vi "FipsAdjacent.vi"() -> (11 "Fips":i32[](array[numeric]))   [LabVIEW 2017] (continued)
\"\t36077\t\"Madison County, NY\"\t36053\n\"Otsego County, NY\"\t36077\t\"Montgomery County, NY\"\t36057\n\"Otsego County, NY\"\t36077\t\"Oneida County, NY\"\t36065\n\"Otsego County, NY\"\t36077\t\"Otsego County, NY\"\t36077\n\"Otsego County, NY\"\t36077\t\"Schoharie County, NY\"\t36095\n\"Putnam County, NY\"\t36079\t\"Fairfield County, CT\"\t09001\n\"Putnam County, NY\"\t36079\t\"Dutchess County, NY\"\t36027\n\"Putnam County, NY\"\t36079\t\"Orange County, NY\"\t36071\n\"Putnam County, NY\"\t36079\t\"Putnam County, NY\"\t36079\n\"Putnam County, NY\"\t36079\t\"Rockland County, NY\"\t36087\n\"Putnam County, NY\"\t36079\t\"Westchester County, NY\"\t36119\n\"Queens County, NY\"\t36081\t\"Monmouth County, NJ\"\t34025\n\"Queens County, NY\"\t36081\t\"Bronx County, NY\"\t36005\n\"Queens County, NY\"\t36081\t\"Kings County, NY\"\t36047\n\"Queens County, NY\"\t36081\t\"Nassau County, NY\"\t36059\n\"Queens County, NY\"\t36081\t\"New York County, NY\"\t36061\n\"Queens County, NY\"\t36081\t\"Queens County, NY\"\t36081\n\"Queens County, NY\"\t36081\t\"Richmond County, NY\"\t36085\n\"Rensselaer County, NY\"\t36083\t\"Berkshire County, MA\"\t25003\n\"Rensselaer County, NY\"\t36083\t\"Albany County, NY\"\t36001\n\"Rensselaer County, NY\"\t36083\t\"Columbia County, NY\"\t36021\n\"Rensselaer County, NY\"\t36083\t\"Greene County, NY\"\t36039\n\"Rensselaer County, NY\"\t36083\t\"Rensselaer County, NY\"\t36083\n\"Rensselaer County, NY\"\t36083\t\"Saratoga County, NY\"\t36091\n\"Rensselaer County, NY\"\t36083\t\"Washington County, NY\"\t36115\n\"Rensselaer County, NY\"\t36083\t\"Bennington County, VT\"\t50003\n\"Richmond County, NY\"\t36085\t\"Hudson County, NJ\"\t34017\n\"Richmond County, NY\"\t36085\t\"Middlesex County, NJ\"\t34023\n\"Richmond County, NY\"\t36085\t\"Monmouth County, NJ\"\t34025\n\"Richmond County, NY\"\t36085\t\"Union County, NJ\"\t34039\n\"Richmond County, NY\"\t36085\t\"Kings County, NY\"\t36047\n\"Richmond County, NY\"\t36085\t\"Queens County, NY\"\t36081\n\"Richmond County, NY\"\t36085\t\"Richmond County, NY\"\t36085\n\"Rockland County, NY\"\t36087\t\"Bergen County, NJ\"\t34003\n\"Rockland County, NY\"\t36087\t\"Passaic County, NJ\"\t34031\n\"Rockland County, NY\"\t36087\t\"Orange County, NY\"\t36071\n\"Rockland County, NY\"\t36087\t\"Putnam County, NY\"\t36079\n\"Rockland County, NY\"\t36087\t\"Rockland County, NY\"\t36087\n\"Rockland County, NY\"\t36087\t\"Westchester County, NY\"\t36119\n\"St. Lawrence County, NY\"\t36089\t\"Franklin County, NY\"\t36033\n\"St. Lawrence County, NY\"\t36089\t\"Hamilton County, NY\"\t36041\n\"St. Lawrence County, NY\"\t36089\t\"Herkimer County, NY\"\t36043\n\"St. Lawrence County, NY\"\t36089\t\"Jefferson County, NY\"\t36045\n\"St. Lawrence County, NY\"\t36089\t\"Lewis County, NY\"\t36049\n\"St. Lawrence County, NY\"\t36089\t\"St. Lawrence County, NY\"\t36089\n\"Saratoga County, NY\"\t36091\t\"Albany County, NY\"\t36001\n\"Saratoga County, NY\"\t36091\t\"Fulton County, NY\"\t36035\n\"Saratoga County, NY\"\t36091\t\"Hamilton County, NY\"\t36041\n\"Saratoga County, NY\"\t36091\t\"Montgomery County, NY\"\t36057\n\"Saratoga County, NY\"\t36091\t\"Rensselaer County, NY\"\t36083\n\"Saratoga County, NY\"\t36091\t\"Saratoga County, NY\"\t36091\n\"Saratoga County, NY\"\t36091\t\"Schenectady County, NY\"\t36093\n\"Saratoga County, NY\"\t36091\t\"Warren County, NY\"\t36113\n\"Saratoga County, NY\"\t36091\t\"Washington County, NY\"\t36115\n\"Schenectady County, NY\"\t36093\t\"Albany County, NY\"\t36001\n\"Schenectady County, NY\"\t36093\t\"Montgomery County, NY\"\t36057\n\"Schenectady County, NY\"\t36093\t\"Saratoga County, NY\"\t36091\n\"Schenectady County, NY\"\t36093\t\"Schenectady County, NY\"\t36093\n\"Schenectady County, NY\"\t36093\t\"Schoharie County, NY\"\t36095\n\"Schoharie County, NY\"\t36095\t\"Albany County, NY\"\t36001\n\"Schoharie County, NY\"\t36095\t\"Delaware County, NY\"\t36025\n\"Schoharie County, NY\"\t36095\t\"Greene County, NY\"\t36039\n\"Schoharie County, NY\"\t36095\t\"Montgomery County, NY\"\t36057\n\"Schoharie County, NY\"\t36095\t\"Otsego County, NY\"\t36077\n\"Schoharie County, NY\"\t36095\t\"Schenectady County, NY\"\t36093\n\"Schoharie County, NY\"\t36095\t\"Schoharie County, NY\"\t36095\n\"Schuyler County, NY\"\t36097\t\"Chemung County, NY\"\t36015\n\"Schuyler County, NY\"\t36097\t\"Schuyler County, NY\"\t36097\n\"Schuyler County, NY\"\t36097\t\"Seneca County, NY\"\t36099\n\"Schuyler County, NY\"\t36097\t\"Steuben County, NY\"\t36101\n\"Schuyler County, NY\"\t36097\t\"Tompkins County, NY\"\t36109\n\"Schuyler County, NY\"\t36097\t\"Yates County, NY\"\t36123\n\"Seneca County, NY\"\t36099\t\"Cayuga County, NY\"\t36011\n\"Seneca County, NY\"\t36099\t\"Ontario County, NY\"\t36069\n\"Seneca County, NY\"\t36099\t\"Schuyler County, NY\"\t36097\n\"Seneca County, NY\"\t36099\t\"Seneca County, NY\"\t36099\n\"Seneca County, NY\"\t36099\t\"Tompkins County, NY\"\t36109\n\"Seneca County, NY\"\t36099\t\"Wayne County, NY\"\t36117\n\"Seneca County, NY\"\t36099\t\"Yates County, NY\"\t36123\n\"Steuben County, NY\"\t36101\t\"Allegany County, NY\"\t36003\n\"Steuben County, NY\"\t36101\t\"Chemung County, NY\"\t36015\n\"Steuben County, NY\"\t36101\t\"Livingston County, NY\"\t36051\n\"Steuben County, NY\"\t36101\t\"Ontario County, NY\"\t36069\n\"Steuben County, NY\"\t36101\t\"Schuyler County, NY\"\t36097\n\"Steuben County, NY\"\t36101\t\"Steuben County, NY\"\t36101\n\"Steuben County, NY\"\t36101\t\"Yates County, NY\"\t36123\n\"Steuben County, NY\"\t36101\t\"Potter County, PA\"\t42105\n\"Steuben County, NY\"\t36101\t\"Tioga County, PA\"\t42117\n\"Suffolk County, NY\"\t36103\t\"Fairfield County, CT\"\t09001\n\"Suffolk County, NY\"\t36103\t\"Middlesex County, CT\"\t09007\n\"Suffolk County, NY\"\t36103\t\"New Haven County, CT\"\t09009\n\"Suffolk County, NY\"\t36103\t\"New London County, CT\"\t09011\n\"Suffolk County, NY\"\t36103\t\"Nassau County, NY\"\t36059\n\"Suffolk County, NY\"\t36103\t\"Suffolk County, NY\"\t36103\n\"Suffolk County, NY\"\t36103\t\"Washington County, RI\"\t44009\n\"Sullivan County, NY\"\t36105\t\"Delaware County, NY\"\t36025\n\"Sullivan County, NY\"\t36105\t\"Orange County, NY\"\t36071\n\"Sullivan County, NY\"\t36105\t\"Sullivan County, NY\"\t36105\n\"Sullivan County, NY\"\t36105\t\"Ulster County, NY\"\t36111\n\"Sullivan County, NY\"\t36105\t\"Pike County, PA\"\t42103\n\"Sullivan County, NY\"\t36105\t\"Wayne County, PA\"\t42127\n\"Tioga County, NY\"\t36107\t\"Broome County, NY\"\t36007\n\"Tioga County, NY\"\t36107\t\"Chemung County, NY\"\t36015\n\"Tioga County, NY\"\t36107\t\"Cortland County, NY\"\t36023\n\"Tioga County, NY\"\t36107\t\"Tioga County, NY\"\t36107\n\"Tioga County, NY\"\t36107\t\"Tompkins County, NY\"\t36109\n\"Tioga County, NY\"\t36107\t\"Bradford County, PA\"\t42015\n\"Tioga County, NY\"\t36107\t\"Susquehanna County, PA\"\t42115\n\"Tompkins County, NY\"\t36109\t\"Cayuga County, NY\"\t36011\n\"Tompkins County, NY\"\t36109\t\"Chemung County, NY\"\t36015\n\"Tompkins County, NY\"\t36109\t\"Cortland County, NY\"\t36023\n\"Tompkins County, NY\"\t36109\t\"Schuyler County, NY\"\t36097\n\"Tompkins County, NY\"\t36109\t\"Seneca County, NY\"\t36099\n\"Tompkins County, NY\"\t36109\t\"Tioga County, NY\"\t36107\n\"Tompkins County, NY\"\t36109\t\"Tompkins County, NY\"\t36109\n\"Ulster County, NY\"\t36111\t\"Columbia County, NY\"\t36021\n\"Ulster County, NY\"\t36111\t\"Delaware County, NY\"\t36025\n\"Ulster County, NY\"\t36111\t\"Dutchess County, NY\"\t36027\n\"Ulster County, NY\"\t36111\t\"Greene County, NY\"\t36039\n\"Ulster County, NY\"\t36111\t\"Orange County, NY\"\t36071\n\"Ulster County, NY\"\t36111\t\"Sullivan County, NY\"\t36105\n\"Ulster County, NY\"\t36111\t\"Ulster County, NY\"\t36111\n\"Warren County, NY\"\t36113\t\"Essex County, NY\"\t36031\n\"Warren County, NY\"\t36113\t\"Hamilton County, NY\"\t36041\n\"Warren County, NY\"\t36113\t\"Saratoga County, NY\"\t36091\n\"Warren County, NY\"\t36113\t\"Warren County, NY\"\t36113\n\"Warren County, NY\"\t36113\t\"Washington County, NY\"\t36115\n\"Washington County, NY\"\t36115\t\"Essex County, NY\"\t36031\n\"Washington County, NY\"\t36115\t\"Rensselaer County, NY\"\t36083\n\"Washington County, NY\"\t36115\t\"Saratoga County, NY\"\t36091\n\"Washington County, NY\"\t36115\t\"Warren County, NY\"\t36113\n\"Washington County, NY\"\t36115\t\"Washington County, NY\"\t36115\n\"Washington County, NY\"\t36115\t\"Addison County, VT\"\t50001\n\"Washington County, NY\"\t36115\t\"Bennington County, VT\"\t50003\n\"Washington County, NY\"\t36115\t\"Rutland County, VT\"\t50021\n\"Wayne County, NY\"\t36117\t\"Cayuga County, NY\"\t36011\n\"Wayne County, NY\"\t36117\t\"Monroe County, NY\"\t36055\n\"Wayne County, NY\"\t36117\t\"Ontario County, NY\"\t36069\n\"Wayne County, NY\"\t36117\t\"Seneca County, NY\"\t36099\n\"Wayne County, NY\"\t36117\t\"Wayne County, NY\"\t36117\n\"Westchester County, NY\"\t36119\t\"Fairfield County, CT\"\t09001\n\"Westchester County, NY\"\t36119\t\"Bergen County, NJ\"\t34003\n\"Westchester County, NY\"\t36119\t\"Bronx County, NY\"\t36005\n\"Westchester County, NY\"\t36119\t\"Nassau County, NY\"\t36059\n\"Westchester County, NY\"\t36119\t\"Putnam County, NY\"\t36079\n\"Westchester County, NY\"\t36119\t\"Rockland County, NY\"\t36087\n\"Westchester County, NY\"\t36119\t\"Westchester County, NY\"\t36119\n\"Wyoming County, NY\"\t36121\t\"Allegany County, NY\"\t36003\n\"Wyoming County, NY\"\t36121\t\"Cattaraugus County, NY\"\t36009\n\"Wyoming County, NY\"\t36121\t\"Erie County, NY\"\t36029\n\"Wyoming County, NY\"\t36121\t\"Genesee County, NY\"\t36037\n\"Wyoming County, NY\"\t36121\t\"Livingston County, NY\"\t36051\n\"Wyoming County, NY\"\t36121\t\"Wyoming County, NY\"\t36121\n\"Yates County, NY\"\t36123\t\"Ontario County, NY\"\t36069\n\"Yates County, NY\"\t36123\t\"Schuyler County, NY\"\t36097\n\"Yates County, NY\"\t36123\t\"Seneca County, NY\"\t36099\n\"Yates County, NY\"\t36123\t\"Steuben County, NY\"\t36101\n\"Yates County, NY\"\t36123\t\"Yates County, NY\"\t36123\n\"Alamance County, NC\"\t37001\t\"Alamance County, NC\"\t37001\n\"Alamance County, NC\"\t37001\t\"Caswell County, NC\"\t37033\n\"Alamance County, NC\"\t37001\t\"Chatham County, NC\"\t37037\n\"Alamance County, NC\"\t37001\t\"Guilford County, NC\"\t37081\n\"Alamance County, NC\"\t37001\t\"Orange County, NC\"\t37135\n\"Alamance County, NC\"\t37001\t\"Randolph County, NC\"\t37151\n\"Alamance County, NC\"\t37001\t\"Rockingham County, NC\"\t37157\n\"Alexander County, NC\"\t37003\t\"Alexander County, NC\"\t37003\n\"Alexander County, NC\"\t37003\t\"Caldwell County, NC\"\t37027\n\"Alexander County, NC\"\t37003\t\"Catawba County, NC\"\t37035\n\"Alexander County, NC\"\t37003\t\"Iredell County, NC\"\t37097\n\"Alexander County, NC\"\t37003\t\"Wilkes County, NC\"\t37193\n\"Alleghany County, NC\"\t37005\t\"Alleghany County, NC\"\t37005\n\"Alleghany County, NC\"\t37005\t\"Ashe County, NC\"\t37009\n\"Alleghany County, NC\"\t37005\t\"Surry County, NC\"\t37171\n\"Alleghany County, NC\"\t37005\t\"Wilkes County, NC\"\t37193\n\"Alleghany County, NC\"\t37005\t\"Grayson County, VA\"\t51077\n\"Anson County, NC\"\t37007\t\"Anson County, NC\"\t37007\n\"Anson County, NC\"\t37007\t\"Montgomery County, NC\"\t37123\n\"Anson County, NC\"\t37007\t\"Richmond County, NC\"\t37153\n\"Anson County, NC\"\t37007\t\"Stanly County, NC\"\t37167\n\"Anson County, NC\"\t37007\t\"Union County, NC\"\t37179\n\"Anson County, NC\"\t37007\t\"Chesterfield County, SC\"\t45025\n\"Anson County, NC\"\t37007\t\"Marlboro County, SC\"\t45069\n\"Ashe County, NC\"\t37009\t\"Alleghany County, NC\"\t37005\n\"Ashe County, NC\"\t37009\t\"Ashe County, NC\"\t37009\n\"Ashe County, NC\"\t37009\t\"Watauga County, NC\"\t37189\n\"Ashe County, NC\"\t37009\t\"Wilkes County, NC\"\t37193\n\"Ashe County, NC\"\t37009\t\"Johnson County, TN\"\t47091\n\"Ashe County, NC\"\t37009\t\"Grayson County, VA\"\t51077\n\"Avery County, NC\"\t37011\t\"Avery County, NC\"\t37011\n\"Avery County, NC\"\t37011\t\"Burke County, NC\"\t37023\n\"Avery County, NC\"\t37011\t\"Caldwell County, NC\"\t37027\n\"Avery County, NC\"\t37011\t\"McDowell County, NC\"\t37111\n\"Avery County, NC\"\t37011\t\"Mitchell County, NC\"\t37121\n\"Avery County, NC\"\t37011\t\"Watauga County, NC\"\t37189\n\"Avery County, NC\"\t37011\t\"Carter County, TN\"\t47019\n\"Avery County, NC\"\t37011\t\"Johnson County, TN\"\t47091\n\"Beaufort County, NC\"\t37013\t\"Beaufort County, NC\"\t37013\n\"Beaufort County, NC\"\t37013\t\"Craven County, NC\"\t37049\n\"Beaufort County, NC\"\t37013\t\"Hyde County, NC\"\t37095\n\"Beaufort County, NC\"\t37013\t\"Martin County, NC\"\t37117\n\"Beaufort County, NC\"\t37013\t\"Pamlico County, NC\"\t37137\n\"Beaufort County, NC\"\t37013\t\"Pitt County, NC\"\t37147\n\"Beaufort County, NC\"\t37013\t\"Washington County, NC\"\t37187\n\"Bertie County, NC\"\t37015\t\"Bertie County, NC\"\t37015\n\"Bertie County, NC\"\t37015\t\"Chowan County, NC\"\t37041\n\"Bertie County, NC\"\t37015\t\"Halifax County, NC\"\t37083\n\"Bertie County, NC\"\t37015\t\"Hertford County, NC\"\t37091\n\"Bertie County, NC\"\t37015\t\"Martin County, NC\"\t37117\n\"Bertie County, NC\"\t37015\t\"Northampton County, NC\"\t37131\n\"Bertie County, NC\"\t37015\t\"Washington County, NC\"\t37187\n\"Bladen County, NC\"\t37017\t\"Bladen County, NC\"\t37017\n\"Bladen County, NC\"\t37017\t\"Columbus County, NC\"\t37047\n\"Bladen County, NC\"\t37017\t\"Cumberland County, NC\"\t37051\n\"Bladen County, NC\"\t37017\t\"Pender County, NC\"\t37141\n\"Bladen County, NC\"\t37017\t\"Robeson County, NC\"\t37155\n\"Bladen County, NC\"\t37017\t\"Sampson County, NC\"\t37163\n\"Brunswick County, NC\"\t37019\t\"Brunswick County, NC\"\t37019\n\"Brunswick County, NC\"\t37019\t\"Columbus County, NC\"\t37047\n\"Brunswick County, NC\"\t37019\t\"New Hanover County, NC\"\t37129\n\"Brunswick County, NC\"\t37019\t\"Pender County, NC\"\t37141\n\"Brunswick County, NC\"\t37019\t\"Horry County, SC\"\t45051\n\"Buncombe County, NC\"\t37021\t\"Buncombe County, NC\"\t37021\n\"Buncombe County, NC\"\t37021\t\"Haywood County, NC\"\t37087\n\"Buncombe County, NC\"\t37021\t\"Henderson County, NC\"\t37089\n\"Buncombe County, NC\"\t37021\t\"McDowell County, NC\"\t37111\n\"Buncombe County, NC\"\t37021\t\"Madison County, NC\"\t37115\n\"Buncombe County, NC\"\t37021\t\"Rutherford County, NC\"\t37161\n\"Buncombe County, NC\"\t37021\t\"Yancey County, NC\"\t37199\n\"Burke County, NC\"\t37023\t\"Avery County, NC\"\t37011\n\"Burke County, NC\"\t37023\t\"Burke County, NC\"\t37023\n\"Burke County, NC\"\t37023\t\"Caldwell County, NC\"\t37027\n\"Burke County, NC\"\t37023\t\"Catawba County, NC\"\t37035\n\"Burke County, NC\"\t37023\t\"Cleveland County, NC\"\t37045\n\"Burke County, NC\"\t37023\t\"Lincoln County, NC\"\t37109\n\"Burke County, NC\"\t37023\t\"McDowell County, NC\"\t37111\n\"Burke County, NC\"\t37023\t\"Rutherford County, NC\"\t37161\n\"Cabarrus County, NC\"\t37025\t\"Cabarrus County, NC\"\t37025\n\"Cabarrus County, NC\"\t37025\t\"Iredell County, NC\"\t37097\n\"Cabarrus County, NC\"\t37025\t\"Mecklenburg County, NC\"\t37119\n\"Cabarrus County, NC\"\t37025\t\"Rowan County, NC\"\t37159\n\"Cabarrus County, NC\"\t37025\t\"Stanly County, NC\"\t37167\n\"Cabarrus County, NC\"\t37025\t\"Union County, NC\"\t37179\n\"Caldwell County, NC\"\t37027\t\"Alexander County, NC\"\t37003\n\"Caldwell County, NC\"\t37027\t\"Avery County, NC\"\t37011\n\"Caldwell County, NC\"\t37027\t\"Burke County, NC\"\t37023\n\"Caldwell County, NC\"\t37027\t\"Caldwell County, NC\"\t37027\n\"Caldwell County, NC\"\t37027\t\"Catawba County, NC\"\t37035\n\"Caldwell County, NC\"\t37027\t\"Watauga County, NC\"\t37189\n\"Caldwell County, NC\"\t37027\t\"Wilkes County, NC\"\t37193\n\"Camden County, NC\"\t37029\t\"Camden County, NC\"\t37029\n\"Camden County, NC\"\t37029\t\"Currituck County, NC\"\t37053\n\"Camden County, NC\"\t37029\t\"Gates County, NC\"\t37073\n\"Camden County, NC\"\t37029\t\"Pasquotank County, NC\"\t37139\n\"Camden County, NC\"\t37029\t\"Tyrrell County, NC\"\t37177\n\"Camden County, NC\"\t37029\t\"Chesapeake city, VA\"\t51550\n\"Camden County, NC\"\t37029\t\"Suffolk city, VA\"\t51800\n\"Carteret County, NC\"\t37031\t\"Carteret County, NC\"\t37031\n\"Carteret County, NC\"\t37031\t\"Craven County, NC\"\t37049\n\"Carteret County, NC\"\t37031\t\"Hyde County, NC\"\t37095\n\"Carteret County, NC\"\t37031\t\"Jones County, NC\"\t37103\n\"Carteret County, NC\"\t37031\t\"Onslow County, NC\"\t37133\n\"Carteret County, NC\"\t37031\t\"Pamlico County, NC\"\t37137\n\"Caswell County, NC\"\t37033\t\"Alamance County, NC\"\t37001\n\"Caswell County, NC\"\t37033\t\"Caswell County, NC\"\t37033\n\"Caswell County, NC\"\t37033\t\"Orange County, NC\"\t37135\n\"Caswell County, NC\"\t37033\t\"Person County, NC\"\t37145\n\"Caswell County, NC\"\t37033\t\"Rockingham County, NC\"\t37157\n\"Caswell County, NC\"\t37033\t\"Halifax County, VA\"\t51083\n\"Caswell County, NC\"\t37033\t\"Pittsylvania County, VA\"\t51143\n\"Caswell County, NC\"\t37033\t\"Danville city, VA\"\t51590\n\"Catawba County, NC\"\t37035\t\"Alexander County, NC\"\t37003\n\"Catawba County, NC\"\t37035\t\"Burke County, NC\"\t37023\n\"Catawba County, NC\"\t37035\t\"Caldwell County, NC\"\t37027\n\"Catawba County, NC\"\t37035\t\"Catawba County, NC\"\t37035\n\"Catawba County, NC\"\t37035\t\"Iredell County, NC\"\t37097\n\"Catawba County, NC\"\t37035\t\"Lincoln County, NC\"\t37109\n\"Chatham County, NC\"\t37037\t\"Alamance County, NC\"\t37001\n\"Chatham County, NC\"\t37037\t\"Chatham County, NC\"\t37037\n\"Chatham County, NC\"\t37037\t\"Durham County, NC\"\t37063\n\"Chatham County, NC\"\t37037\t\"Harnett County, NC\"\t37085\n\"Chatham County, NC\"\t37037\t\"Lee County, NC\"\t37105\n\"Chatham County, NC\"\t37037\t\"Moore County, NC\"\t37125\n\"Chatham County, NC\"\t37037\t\"Orange County, NC\"\t37135\n\"Chatham County, NC\"\t37037\t\"Randolph County, NC\"\t37151\n\"Chatham County, NC\"\t37037\t\"Wake County, NC\"\t37183\n\"Cherokee County, NC\"\t37039\t\"Fannin County, GA\"\t13111\n\"Cherokee County, NC\"\t37039\t\"Union County, GA\"\t13291\n\"Cherokee County, NC\"\t37039\t\"Cherokee County, NC\"\t37039\n\"Cherokee County, NC\"\t37039\t\"Clay County, NC\"\t37043\n\"Cherokee County, NC\"\t37039\t\"Graham County, NC\"\t37075\n\"Cherokee County, NC\"\t37039\t\"Macon County, NC\"\t37113\n\"Cherokee County, NC\"\t37039\t\"Monroe County, TN\"\t47123\n\"Cherokee County, NC\"\t37039\t\"Polk County, TN\"\t47139\n\"Chowan County, NC\"\t37041\t\"Bertie County, NC\"\t37015\n\"Chowan County, NC\"\t37041\t\"Chowan County, NC\"\t37041\n\"Chowan County, NC\"\t37041\t\"Gates County, NC\"\t37073\n\"Chowan County, NC\"\t37041\t\"Hertford County, NC\"\t37091\n\"Chowan County, NC\"\t37041\t\"Perquimans County, NC\"\t37143\n\"Chowan County, NC\"\t37041\t\"Washington County, NC\"\t37187\n\"Clay County, NC\"\t37043\t\"Rabun County, GA\"\t13241\n\"Clay County, NC\"\t37043\t\"Towns County, GA\"\t13281\n\"Clay County, NC\"\t37043\t\"Union County, GA\"\t13291\n\"Clay County, NC\"\t37043\t\"Cherokee County, NC\"\t37039\n\"Clay County, NC\"\t37043\t\"Clay County, NC\"\t37043\n\"Clay County, NC\"\t37043\t\"Macon County, NC\"\t37113\n\"Cleveland County, NC\"\t37045\t\"Burke County, NC\"\t37023\n\"Cleveland County, NC\"\t37045\t\"Cleveland County, NC\"\t37045\n\"Cleveland County, NC\"\t37045\t\"Gaston County, NC\"\t37071\n\"Cleveland County, NC\"\t37045\t\"Lincoln County, NC\"\t37109\n\"Cleveland County, NC\"\t37045\t\"Rutherford County, NC\"\t37161\n\"Cleveland County, NC\"\t37045\t\"Cherokee County, SC\"\t45021\n\"Cleveland County, NC\"\t37045\t\"York County, SC\"\t45091\n\"Columbus County, NC\"\t37047\t\"Bladen County, NC\"\t37017\n\"Columbus County, NC\"\t37047\t\"Brunswick County, NC\"\t37019\n\"Columbus County, NC\"\t37047\t\"Columbus County, NC\"\t37047\n\"Columbus County, NC\"\t37047\t\"Pender County, NC\"\t37141\n\"Columbus County, NC\"\t37047\t\"Robeson County, NC\"\t37155\n\"Columbus County, NC\"\t37047\t\"Dillon County, SC\"\t45033\n\"Columbus County, NC\"\t37047\t\"Horry County, SC\"\t45051\n\"Craven County, NC\"\t37049\t\"Beaufort County, NC\"\t37013\n\"Craven County, NC\"\t37049\t\"Carteret County, NC\"\t37031\n\"Craven County, NC\"\t37049\t\"Craven County, NC\"\t37049\n\"Craven County, NC\"\t37049\t\"Jones County, NC\"\t37103\n\"Craven County, NC\"\t37049\t\"Lenoir County, NC\"\t37107\n\"Craven County, NC\"\t37049\t\"Pamlico County, NC\"\t37137\n\"Craven County, NC\"\t37049\t\"Pitt County, NC\"\t37147\n\"Cumberland County, NC\"\t37051\t\"Bladen County, NC\"\t37017\n\"Cumberland County, NC\"\t37051\t\"Cumberland County, NC\"\t37051\n\"Cumberland County, NC\"\t37051\t\"Harnett County, NC\"\t37085\n\"Cumberland County, NC\"\t37051\t\"Hoke County, NC\"\t37093\n\"Cumberland County, NC\"\t37051\t\"Moore County, NC\"\t37125\n\"Cumberland County, NC\"\t37051\t\"Robeson County, NC\"\t37155\n\"Cumberland County, NC\"\t37051\t\"Sampson County, NC\"\t37163\n\"Currituck County, NC\"\t37053\t\"Camden County, NC\"\t37029\n\"Currituck County, NC\"\t37053\t\"Currituck County, NC\"\t37053\n\"Currituck County, NC\"\t37053\t\"Dare County, NC\"\t37055\n\"Currituck County, NC\"\t37053\t\"Tyrrell County, NC\"\t37177\n\"Currituck County, NC\"\t37053\t\"Chesapeake city, VA\"\t51550\n\"Currituck County, NC\"\t37053\t\"Virginia Beach city, VA\"\t51810\n\"Dare County, NC\"\t37055\t\"Currituck County, NC\"\t37053\n\"Dare County, NC\"\t37055\t\"Dare County, NC\"\t37055\n\"Dare County, NC\"\t37055\t\"Hyde County, NC\"\t37095\n\"Dare County, NC\"\t37055\t\"Tyrrell County, NC\"\t37177\n\"Davidson County, NC\"\t37057\t\"Davidson County, NC\"\t37057\n\"Davidson County, NC\"\t37057\t\"Davie County, NC\"\t37059\n\"Davidson County, NC\"\t37057\t\"Forsyth County, NC\"\t37067\n\"Davidson County, NC\"\t37057\t\"Guilford County, NC\"\t37081\n\"Davidson County, NC\"\t37057\t\"Montgomery County, NC\"\t37123\n\"Davidson County, NC\"\t37057\t\"Randolph County, NC\"\t37151\n\"Davidson County, NC\"\t37057\t\"Rowan County, NC\"\t37159\n\"Davidson County, NC\"\t37057\t\"Stanly County, NC\"\t37167\n\"Davie County, NC\"\t37059\t\"Davidson County, NC\"\t37057\n\"Davie County, NC\"\t37059\t\"Davie County, NC\"\t37059\n\"Davie County, NC\"\t37059\t\"Forsyth County, NC\"\t37067\n\"Davie County, NC\"\t37059\t\"Iredell County, NC\"\t37097\n\"Davie County, NC\"\t37059\t\"Rowan County, NC\"\t37159\n\"Davie County, NC\"\t37059\t\"Yadkin County, NC\"\t37197\n\"Duplin County, NC\"\t37061\t\"Duplin County, NC\"\t37061\n\"Duplin County, NC\"\t37061\t\"Jones County, NC\"\t37103\n\"Duplin County, NC\"\t37061\t\"Lenoir County, NC\"\t37107\n\"Duplin County, NC\"\t37061\t\"Onslow County, NC\"\t37133\n\"Duplin County, NC\"\t37061\t\"Pender County, NC\"\t37141\n\"Duplin County, NC\"\t37061\t\"Sampson County, NC\"\t37163\n\"Duplin County, NC\"\t37061\t\"Wayne County, NC\"\t37191\n\"Durham County, NC\"\t37063\t\"Chatham County, NC\"\t37037\n\"Durham County, NC\"\t37063\t\"Durham County, NC\"\t37063\n\"Durham County, NC\"\t37063\t\"Granville County, NC\"\t37077\n\"Durham County, NC\"\t37063\t\"Orange County, NC\"\t37135\n\"Durham County, NC\"\t37063\t\"Person County, NC\"\t37145\n\"Durham County, NC\"\t37063\t\"Wake County, NC\"\t37183\n\"Edgecombe County, NC\"\t37065\t\"Edgecombe County, NC\"\t37065\n\"Edgecombe County, NC\"\t37065\t\"Halifax County, NC\"\t37083\n\"Edgecombe County, NC\"\t37065\t\"Martin County, NC\"\t37117\n\"Edgecombe County, NC\"\t37065\t\"Nash County, NC\"\t37127\n\"Edgecombe County, NC\"\t37065\t\"Pitt County, NC\"\t37147\n\"Edgecombe County, NC\"\t37065\t\"Wilson County, NC\"\t37195\n\"Forsyth County, NC\"\t37067\t\"Davidson County, NC\"\t37057\n\"Forsyth County, NC\"\t37067\t\"Davie County, NC\"\t37059\n\"Forsyth County, NC\"\t37067\t\"Forsyth County, NC\"\t37067\n\"Forsyth County, NC\"\t37067\t\"Guilford County, NC\"\t37081\n\"Forsyth County, NC\"\t37067\t\"Rockingham County, NC\"\t37157\n\"Forsyth County, NC\"\t37067\t\"Stokes County, NC\"\t37169\n\"Forsyth County, NC\"\t37067\t\"Surry County, NC\"\t37171\n\"Forsyth County, NC\"\t37067\t\"Yadkin County, NC\"\t37197\n\"Franklin County, NC\"\t37069\t\"Franklin County, NC\"\t37069\n\"Franklin County, NC\"\t37069\t\"Granville County, NC\"\t37077\n\"Franklin County, NC\"\t37069\t\"Halifax County, NC\"\t37083\n\"Franklin County, NC\"\t37069\t\"Johnston County, NC\"\t37101\n\"Franklin County, NC\"\t37069\t\"Nash County, NC\"\t37127\n\"Franklin County, NC\"\t37069\t\"Vance County, NC\"\t37181\n\"Franklin County, NC\"\t37069\t\"Wake County, NC\"\t37183\n\"Franklin County, NC\"\t37069\t\"Warren County, NC\"\t37185\n\"Gaston County, NC\"\t37071\t\"Cleveland County, NC\"\t37045\n\"Gaston County, NC\"\t37071\t\"Gaston County, NC\"\t37071\n\"Gaston County, NC\"\t37071\t\"Lincoln County, NC\"\t37109\n\"Gaston County, NC\"\t37071\t\"Mecklenburg County, NC\"\t37119\n\"Gaston County, NC\"\t37071\t\"York County, SC\"\t45091\n\"Gates County, NC\"\t37073\t\"Camden County, NC\"\t37029\n\"Gates County, NC\"\t37073\t\"Chowan County, NC\"\t37041\n\"Gates County, NC\"\t37073\t\"Gates County, NC\"\t37073\n\"Gates County, NC\"\t37073\t\"Hertford County, NC\"\t37091\n\"Gates County, NC\"\t37073\t\"Pasquotank County, NC\"\t37139\n\"Gates County, NC\"\t37073\t\"Perquimans County, NC\"\t37143\n\"Gates County, NC\"\t37073\t\"Southampton County, VA\"\t51175\n\"Gates County, NC\"\t37073\t\"Suffolk city, VA\"\t51800\n\"Graham County, NC\"\t37075\t\"Cherokee County, NC\"\t37039\n\"Graham County, NC\"\t37075\t\"Graham County, NC\"\t37075\n\"Graham County, NC\"\t37075\t\"Macon County, NC\"\t37113\n\"Graham County, NC\"\t37075\t\"Swain County, NC\"\t37173\n\"Graham County, NC\"\t37075\t\"Blount County, TN\"\t47009\n\"Graham County, NC\"\t37075\t\"Monroe County, TN\"\t47123\n\"Granville County, NC\"\t37077\t\"Durham County, NC\"\t37063\n\"Granville County, NC\"\t37077\t\"Franklin County, NC\"\t37069\n\"Granville County, NC\"\t37077\t\"Granville County, NC\"\t37077\n\"Granville County, NC\"\t37077\t\"Person County, NC\"\t37145\n\"Granville County, NC\"\t37077\t\"Vance County, NC\"\t37181\n\"Granville County, NC\"\t37077\t\"Wake County, NC\"\t37183\n\"Granville County, NC\"\t37077\t\"Halifax County, VA\"\t51083\n\"Granville County, NC\"\t37077\t\"Mecklenburg County, VA\"\t51117\n\"Greene County, NC\"\t37079\t\"Greene County, NC\"\t37079\n\"Greene County, NC\"\t37079\t\"Lenoir County, NC\"\t37107\n\"Greene County, NC\"\t37079\t\"Pitt County, NC\"\t37147\n\"Greene County, NC\"\t37079\t\"Wayne County, NC\"\t37191\n\"Greene County, NC\"\t37079\t\"Wilson County, NC\"\t37195\n\"Guilford County, NC\"\t37081\t\"Alamance County, NC\"\t37001\n\"Guilford County, NC\"\t37081\t\"Davidson County, NC\"\t37057\n\"Guilford County, NC\"\t37081\t\"Forsyth County, NC\"\t37067\n\"Guilford County, NC\"\t37081\t\"Guilford County, NC\"\t37081\n\"Guilford County, NC\"\t37081\t\"Randolph County, NC\"\t37151\n\"Guilford County, NC\"\t37081\t\"Rockingham County, NC\"\t37157\n\"Guilford County, NC\"\t37081\t\"Stokes County, NC\"\t37169\n\"Halifax County, NC\"\t37083\t\"Bertie County, NC\"\t37015\n\"Halifax County, NC\"\t37083\t\"Edgecombe County, NC\"\t37065\n\"Halifax County, NC\"\t37083\t\"Franklin County, NC\"\t37069\n\"Halifax County, NC\"\t37083\t\"Halifax County, NC\"\t37083\n\"Halifax County, NC\"\t37083\t\"Martin County, NC\"\t37117\n\"Halifax County, NC\"\t37083\t\"Nash County, NC\"\t37127\n\"Halifax County, NC\"\t37083\t\"Northampton County, NC\"\t37131\n\"Halifax County, NC\"\t37083\t\"Warren County, NC\"\t37185\n\"Harnett County, NC\"\t37085\t\"Chatham County, NC\"\t37037\n\"Harnett County, NC\"\t37085\t\"Cumberland County, NC\"\t37051\n\"Harnett County, NC\"\t37085\t\"Harnett County, NC\"\t37085\n\"Harnett County, NC\"\t37085\t\"Johnston County, NC\"\t37101\n\"Harnett County, NC\"\t37085\t\"Lee County, NC\"\t37105\n\"Harnett County, NC\"\t37085\t\"Moore County, NC\"\t37125\n\"Harnett County, NC\"\t37085\t\"Sampson County, NC\"\t37163\n\"Harnett County, NC\"\t37085\t\"Wake County, NC\"\t37183\n\"Haywood County, NC\"\t37087\t\"Buncombe County, NC\"\t37021\n\"Haywood County, NC\"\t37087\t\"Haywood County, NC\"\t37087\n\"Haywood County, NC\"\t37087\t\"Henderson County, NC\"\t37089\n\"Haywood County, NC\"\t37087\t\"Jackson County, NC\"\t37099\n\"Haywood County, NC\"\t37087\t\"Madison County, NC\"\t37115\n\"Haywood County, NC\"\t37087\t\"Swain County, NC\"\t37173\n\"Haywood County, NC\"\t37087\t\"Transylvania County, NC\"\t37175\n\"Haywood County, NC\"\t37087\t\"Cocke County, TN\"\t47029\n\"Haywood County, NC\"\t37087\t\"Sevier County, TN\"\t47155\n\"Henderson County, NC\"\t37089\t\"Buncombe County, NC\"\t37021\n\"Henderson County, NC\"\t37089\t\"Haywood County, NC\"\t37087\n\"Henderson County, NC\"\t37089\t\"Henderson County, NC\"\t37089\n\"Henderson County, NC\"\t37089\t\"Polk County, NC\"\t37149\n\"Henderson County, NC\"\t37089\t\"Rutherford County, NC\"\t37161\n\"Henderson County, NC\"\t37089\t\"Transylvania County, NC\"\t37175\n\"Henderson County, NC\"\t37089\t\"Greenville County, SC\"\t45045\n\"Hertford County, NC\"\t37091\t\"Bertie County, NC\"\t37015\n\"Hertford County, NC\"\t37091\t\"Chowan County, NC\"\t37041\n\"Hertford County, NC\"\t37091\t\"Gates County, NC\"\t37073\n\"Hertford County, NC\"\t37091\t\"Hertford County, NC\"\t37091\n\"Hertford County, NC\"\t37091\t\"Northampton County, NC\"\t37131\n\"Hertford County, NC\"\t37091\t\"Southampton County, VA\"\t51175\n\"Hoke County, NC\"\t37093\t\"Cumberland County, NC\"\t37051\n\"Hoke County, NC\"\t37093\t\"Hoke County, NC\"\t37093\n\"Hoke County, NC\"\t37093\t\"Moore County, NC\"\t37125\n\"Hoke County, NC\"\t37093\t\"Richmond County, NC\"\t37153\n\"Hoke County, NC\"\t37093\t\"Robeson County, NC\"\t37155\n\"Hoke County, NC\"\t37093\t\"Scotland County, NC\"\t37165\n\"Hyde County, NC\"\t37095\t\"Beaufort County, NC\"\t37013\n\"Hyde County, NC\"\t37095\t\"Carteret County, NC\"\t37031\n\"Hyde County, NC\"\t37095\t\"Dare County, NC\"\t37055\n\"Hyde County, NC\"\t37095\t\"Hyde County, NC\"\t37095\n\"Hyde County, NC\"\t37095\t\"Pamlico County, NC\"\t37137\n\"Hyde County, NC\"\t37095\t\"Tyrrell County, NC\"\t37177\n\"Hyde County, NC\"\t37095\t\"Washington County, NC\"\t37187\n\"Iredell County, NC\"\t37097\t\"Alexander County, NC\"\t37003\n\"Iredell County, NC\"\t37097\t\"Cabarrus County, NC\"\t37025\n\"Iredell County, NC\"\t37097\t\"Catawba County, NC\"\t37035\n\"Iredell County, NC\"\t37097\t\"Davie County, NC\"\t37059\n\"Iredell County, NC\"\t37097\t\"Iredell County, NC\"\t37097\n\"Iredell County, NC\"\t37097\t\"Lincoln County, NC\"\t37109\n\"Iredell County, NC\"\t37097\t\"Mecklenburg County, NC\"\t37119\n\"Iredell County, NC\"\t37097\t\"Rowan County, NC\"\t37159\n\"Iredell County, NC\"\t37097\t\"Wilkes County, NC\"\t37193\n\"Iredell County, NC\"\t37097\t\"Yadkin County, NC\"\t37197\n\"Jackson County, NC\"\t37099\t\"Rabun County, GA\"\t13241\n\"Jackson County, NC\"\t37099\t\"Haywood County, NC\"\t37087\n\"Jackson County, NC\"\t37099\t\"Jackson County, NC\"\t37099\n\"Jackson County, NC\"\t37099\t\"Macon County, NC\"\t37113\n\"Jackson County, NC\"\t37099\t\"Swain County, NC\"\t37173\n\"Jackson County, NC\"\t37099\t\"Transylvania County, NC\"\t37175\n\"Jackson County, NC\"\t37099\t\"Oconee County, SC\"\t45073\n\"Johnston County, NC\"\t37101\t\"Franklin County, NC\"\t37069\n\"Johnston County, NC\"\t37101\t\"Harnett County, NC\"\t37085\n\"Johnston County, NC\"\t37101\t\"Johnston County, NC\"\t37101\n\"Johnston County, NC\"\t37101\t\"Nash County, NC\"\t37127\n\"Johnston County, NC\"\t37101\t\"Sampson County, NC\"\t37163\n\"Johnston County, NC\"\t37101\t\"Wake County, NC\"\t37183\n\"Johnston County, NC\"\t37101\t\"Wayne County, NC\"\t37191\n\"Johnston County, NC\"\t37101\t\"Wilson County, NC\"\t37195\n\"Jones County, NC\"\t37103\t\"Carteret County, NC\"\t37031\n\"Jones County, NC\"\t37103\t\"Craven County, NC\"\t37049\n\"Jones County, NC\"\t37103\t\"Duplin County, NC\"\t37061\n\"Jones County, NC\"\t37103\t\"Jones County, NC\"\t37103\n\"Jones County, NC\"\t37103\t\"Lenoir County, NC\"\t37107\n\"Jones County, NC\"\t37103\t\"Onslow County, NC\"\t37133\n\"Lee County, NC\"\t37105\t\"Chatham County, NC\"\t37037\n\"Lee County, NC\"\t37105\t\"Harnett County, NC\"\t37085\n\"Lee County, NC\"\t37105\t\"Lee County, NC\"\t37105\n\"Lee County, NC\"\t37105\t\"Moore County, NC\"\t37125\n\"Lenoir County, NC\"\t37107\t\"Craven County, NC\"\t37049\n\"Lenoir County, NC\"\t37107\t\"Duplin County, NC\"\t37061\n\"Lenoir County, NC\"\t37107\t\"Greene County, NC\"\t37079\n\"Lenoir County, NC\"\t37107\t\"Jones County, NC\"\t37103\n\"Lenoir County, NC\"\t37107\t\"Lenoir County, NC\"\t37107\n\"Lenoir County, NC\"\t37107\t\"Pitt County, NC\"\t37147\n\"Lenoir County, NC\"\t37107\t\"Wayne County, NC\"\t37191\n\"Lincoln County, NC\"\t37109\t\"Burke County, NC\"\t37023\n\"Lincoln County, NC\"\t37109\t\"Catawba County, NC\"\t37035\n\"Lincoln County, NC\"\t37109\t\"Cleveland County, NC\"\t37045\n\"Lincoln County, NC\"\t37109\t\"Gaston County, NC\"\t37071\n\"Lincoln County, NC\"\t37109\t\"Iredell County, NC\"\t37097\n\"Lincoln County, NC\"\t37109\t\"Lincoln County, NC\"\t37109\n\"Lincoln County, NC\"\t37109\t\"Mecklenburg County, NC\"\t37119\n\"McDowell County, NC\"\t37111\t\"Avery County, NC\"\t37011\n\"McDowell County, NC\"\t37111\t\"Buncombe County, NC\"\t37021\n\"McDowell County, NC\"\t37111\t\"Burke County, NC\"\t37023\n\"McDowell County, NC\"\t37111\t\"McDowell County, NC\"\t37111\n\"McDowell County, NC\"\t37111\t\"Mitchell County, NC\"\t37121\n\"McDowell County, NC\"\t37111\t\"Rutherford County, NC\"\t37161\n\"McDowell County, NC\"\t37111\t\"Yancey County, NC\"\t37199\n\"Macon County, NC\"\t37113\t\"Rabun County, GA\"\t13241\n\"Macon County, NC\"\t37113\t\"Cherokee County, NC\"\t37039\n\"Macon County, NC\"\t37113\t\"Clay County, NC\"\t37043\n\"Macon County, NC\"\t37113\t\"Graham County, NC\"\t37075\n\"Macon County, NC\"\t37113\t\"Jackson County, NC\"\t37099\n\"Macon County, NC\"\t37113\t\"Macon County, NC\"\t37113\n\"Macon County, NC\"\t37113\t\"Swain County, NC\"\t37173\n\"Macon County, NC\"\t37113\t\"Oconee County, SC\"\t45073\n\"Madison County, NC\"\t37115\t\"Buncombe County, NC\"\t37021\n\"Madison County, NC\"\t37115\t\"Haywood County, NC\"\t37087\n\"Madison County, NC\"\t37115\t\"Madison County, NC\"\t37115\n\"Madison County, NC\"\t37115\t\"Yancey County, NC\"\t37199\n\"Madison County, NC\"\t37115\t\"Cocke County, TN\"\t47029\n\"Madison County, NC\"\t37115\t\"Greene County, TN\"\t47059\n\"Madison County, NC\"\t37115\t\"Unicoi County, TN\"\t47171\n\"Martin County, NC\"\t37117\t\"Beaufort County, NC\"\t37013\n\"Martin County, NC\"\t37117\t\"Bertie County, NC\"\t37015\n\"Martin County, NC\"\t37117\t\"Edgecombe County, NC\"\t37065\n\"Martin County, NC\"\t37117\t\"Halifax County, NC\"\t37083\n\"Martin County, NC\"\t37117\t\"Martin County, NC\"\t37117\n\"Martin County, NC\"\t37117\t\"Pitt County, NC\"\t37147\n\"Martin County, NC\"\t37117\t\"Washington County, NC\"\t37187\n\"Mecklenburg County, NC\"\t37119\t\"Cabarrus County, NC\"\t37025\n\"Mecklenburg County, NC\"\t37119\t\"Gaston County, NC\"\t37071\n\"Mecklenburg County, NC\"\t37119\t\"Iredell County, NC\"\t37097\n\"Mecklenburg County, NC\"\t37119\t\"Lincoln County, NC\"\t37109\n\"Mecklenburg County, NC\"\t37119\t\"Mecklenburg County, NC\"\t37119\n\"Mecklenburg County, NC\"\t37119\t\"Union County, NC\"\t37179\n\"Mecklenburg County, NC\"\t37119\t\"Lancaster County, SC\"\t45057\n\"Mecklenburg County, NC\"\t37119\t\"York County, SC\"\t45091\n\"Mitchell County, NC\"\t37121\t\"Avery County, NC\"\t37011\n\"Mitchell County, NC\"\t37121\t\"McDowell County, NC\"\t37111\n\"Mitchell County, NC\"\t37121\t\"Mitchell County, NC\"\t37121\n\"Mitchell County, NC\"\t37121\t\"Yancey County, NC\"\t37199\n\"Mitchell County, NC\"\t37121\t\"Carter County, TN\"\t47019\n\"Mitchell County, NC\"\t37121\t\"Unicoi County, TN\"\t47171\n\"Montgomery County, NC\"\t37123\t\"Anson County, NC\"\t37007\n\"Montgomery County, NC\"\t37123\t\"Davidson County, NC\"\t37057\n\"Montgomery County, NC\"\t37123\t\"Montgomery County, NC\"\t37123\n\"Montgomery County, NC\"\t37123\t\"Moore County, NC\"\t37125\n\"Montgomery County, NC\"\t37123\t\"Randolph County, NC\"\t37151\n\"Montgomery County, NC\"\t37123\t\"Richmond County, NC\"\t37153\n\"Montgomery County, NC\"\t37123\t\"Rowan County, NC\"\t37159\n\"Montgomery County, NC\"\t37123\t\"Stanly County, NC\"\t37167\n\"Moore County, NC\"\t37125\t\"Chatham County, NC\"\t37037\n\"Moore County, NC\"\t37125\t\"Cumberland County, NC\"\t37051\n\"Moore County, NC\"\t37125\t\"Harnett County, NC\"\t37085\n\"Moore County, NC\"\t37125\t\"Hoke County, NC\"\t37093\n\"Moore County, NC\"\t37125\t\"Lee County, NC\"\t37105\n\"Moore County, NC\"\t37125\t\"Montgomery County, NC\"\t37123\n\"Moore County, NC\"\t37125\t\"Moore County, NC\"\t37125\n\"Moore County, NC\"\t37125\t\"Randolph County, NC\"\t37151\n\"Moore County, NC\"\t37125\t\"Richmond County, NC\"\t37153\n\"Moore County, NC\"\t37125\t\"Scotland County, NC\"\t37165\n\"Nash County, NC\"\t37127\t\"Edgecombe County, NC\"\t37065\n\"Nash County, NC\"\t37127\t\"Franklin County, NC\"\t37069\n\"Nash County, NC\"\t37127\t\"Halifax County, NC\"\t37083\n\"Nash County, NC\"\t37127\t\"Johnston County, NC\"\t37101\n\"Nash County, NC\"\t37127\t\"Nash County, NC\"\t37127\n\"Nash County, NC\"\t37127\t\"Wake County, NC\"\t37183\n\"Nash County, NC\"\t37127\t\"Warren County, NC\"\t37185\n\"Nash County, NC\"\t37127\t\"Wilson County, NC\"\t37195\n\"New Hanover County, NC\"\t37129\t\"Brunswick County, NC\"\t37019\n\"New Hanover County, NC\"\t37129\t\"New Hanover County, NC\"\t37129\n\"New Hanover County, NC\"\t37129\t\"Pender County, NC\"\t37141\n\"Northampton County, NC\"\t37131\t\"Bertie County, NC\"\t37015\n\"Northampton County, NC\"\t37131\t\"Halifax County, NC\"\t37083\n\"Northampton County, NC\"\t37131\t\"Hertford County, NC\"\t37091\n\"Northampton County, NC\"\t37131\t\"Northampton County, NC\"\t37131\n\"Northampton County, NC\"\t37131\t\"Warren County, NC\"\t37185\n\"Northampton County, NC\"\t37131\t\"Brunswick County, VA\"\t51025\n\"Northampton County, NC\"\t37131\t\"Greensville County, VA\"\t51081\n\"Northampton County, NC\"\t37131\t\"Southampton County, VA\"\t51175\n\"Onslow County, NC\"\t37133\t\"Carteret County, NC\"\t37031\n\"Onslow County, NC\"\t37133\t\"Duplin County, NC\"\t37061\n\"Onslow County, NC\"\t37133\t\"Jones County, NC\"\t37103\n\"Onslow County, NC\"\t37133\t\"Onslow County, NC\"\t37133\n\"Onslow County, NC\"\t37133\t\"Pender County, NC\"\t37141\n\"Orange County, NC\"\t37135\t\"Alamance County, NC\"\t37001\n\"Orange County, NC\"\t37135\t\"Caswell County, NC\"\t37033\n\"Orange County, NC\"\t37135\t\"Chatham County, NC\"\t37037\n\"Orange County, NC\"\t37135\t\"Durham County, NC\"\t37063\n\"Orange County, NC\"\t37135\t\"Orange County, NC\"\t37135\n\"Orange County, NC\"\t37135\t\"Person County, NC\"\t37145\n\"Pamlico County, NC\"\t37137\t\"Beaufort County, NC\"\t37013\n\"Pamlico County, NC\"\t37137\t\"Carteret County, NC\"\t37031\n\"Pamlico County, NC\"\t37137\t\"Craven County, NC\"\t37049\n\"Pamlico County, NC\"\t37137\t\"Hyde County, NC\"\t37095\n\"Pamlico County, NC\"\t37137\t\"Pamlico County, NC\"\t37137\n\"Pasquotank County, NC\"\t37139\t\"Camden County, NC\"\t37029\n\"Pasquotank County, NC\"\t37139\t\"Gates County, NC\"\t37073\n\"Pasquotank County, NC\"\t37139\t\"Pasquotank County, NC\"\t37139\n\"Pasquotank County, NC\"\t37139\t\"Perquimans County, NC\"\t37143\n\"Pasquotank County, NC\"\t37139\t\"Tyrrell County, NC\"\t37177\n\"Pender County, NC\"\t37141\t\"Bladen County, NC\"\t37017\n\"Pender County, NC\"\t37141\t\"Brunswick County, NC\"\t37019\n\"Pender County, NC\"\t37141\t\"Columbus County, NC\"\t37047\n\"Pender County, NC\"\t37141\t\"Duplin County, NC\"\t37061\n\"Pender County, NC\"\t37141\t\"New Hanover County, NC\"\t37129\n\"Pender County, NC\"\t37141\t\"Onslow County, NC\"\t37133\n\"Pender County, NC\"\t37141\t\"Pender County, NC\"\t37141\n\"Pender County, NC\"\t37141\t\"Sampson County, NC\"\t37163\n\"Perquimans County, NC\"\t37143\t\"Chowan County, NC\"\t37041\n\"Perquimans County, NC\"\t37143\t\"Gates County, NC\"\t37073\n\"Perquimans County, NC\"\t37143\t\"Pasquotank County, NC\"\t37139\n\"Perquimans County, NC\"\t37143\t
